vi "LIA Example FPGA_v1.vi"() -> ()   [LabVIEW 2017]
uses:
  <instrlib>/_niInstr/Streaming/v1/Common/Stream State.ctl
  <instrlib>/_niInstr/Data Trigger/v1/Shared/Public/Edge Configuration FXP(+-,18,1).ctl
  <instrlib>/_niInstr/Data Trigger/v1/Shared/Public/Edge Configuration Trigger Slope.ctl
  <vilib>/Platform/TimedLoop/XDataNode/timing_clust.ctl
  <vilib>/Platform/TimedLoop/XDataNode/nitl_modes.ctl
  <vilib>/Platform/TimedLoop/XDataNode/wakeup.ctl
  <instrlib>/_niInstr/DSP/v1/Shared/Public/IQ Data.ctl
  <vilib>/rvi/Emulation/niFpgaSctlEmulationGetInTimedLoop.vi
  <vilib>/rvi/Emulation/niFpgaEmulationReportErrorSimple.vi
  <vilib>/rvi/Emulation/niFpgaGetClockAttributes.vi
  <vilib>/rvi/Emulation/niFpgaCriticalErrorInLSC.vi
  <instrlib>/_niInstr/DSP/v1/FPGA/Public/Sub VIs/Frequency Shift/Frequency Shift - 1 spc.vi
  <instrlib>/_niInstr/DSP/v1/FPGA/Public/Sub VIs/Fractional Decimator/Fractional Decimator - 1 spc - 2x oc.vi
  <userlib>/_NI Noise Generation IP/FPGA/Public/Low Level/AWGN FXP23x2.vi
  <instrlib>/_niInstr/DSP/v1/FPGA/Public/Sub VIs/Frequency Shift/Frequency Shift - 2 spc.vi
  <vilib>/rvi/eio/common/nirviEmuTemplateMethod_errors.vi
  <vilib>/Platform/TimedLoop/XDataNode/XDataNode.xnode
  <instrlib>/_niInstr/DSP/v1/Xnodes/Public/Frequency Shift/niInstr DSP v1 Frequency Shift FPGA.xnode
  <vilib>/rvi/FXPMathLib/FxpMul/XNode/nifxpmath_Multiplier.xnode
  <vilib>/rvi/FXPMathLib/FxpAdd/XNode/nifxpmath_Add.xnode
  <vilib>/eio/EIONode/EIONode.xnode
  <vilib>/Platform/TimedLoop/XDataNode/XDNodeRunTimeDep.lvlib
  <instrlib>/_niInstr/Basic Elements/v1/FPGA/niInstr Basic Elements v1 FPGA.lvlib
  <instrlib>/_niInstr/DSP/v1/Shared/niInstr DSP v1 Shared.lvlib
  <instrlib>/_niInstr/DSP/v1/FPGA/niInstr DSP v1 FPGA.lvlib
  lib/fpga/Lock-In Amplifier Example FPGA.lvlib
  <instrlib>/_niInstr/Streaming/v1/Common/niInstr Streaming v1 Common.lvlib
  <userlib>/_NI Noise Generation IP/FPGA/NI Noise Generation IP FPGA v2.lvlib
  <vilib>/rvi/FXPMathLib/sim/FxpSim.dll
  <instrlib>/_niInstr/Data Trigger/v1/Shared/niInstr Data Trigger v1 Shared.lvlib
panel:
  in  "Decimator":enum16{"CIC", "FIR", "Bypassed"}(ring)
  in  "output sample rate":fxp<+,48,1>=0.0009999999999976694
  in  "pll.digital config 1":T1
  in  "pll.digital config 0":T1
  in  "pll.m 0":i8
  in  "pll.m 1":i8
  in  "pll.q 1":fxp<+,48,0>
  in  "pll.q 0":fxp<+,48,0>
  in  "lock-in.enable 3":bool
  in  "lock-in.enable 2":bool
  in  "lock-in.enable 1":bool
  in  "lock-in.carrier 3":fxp<+/-,48,0>
  in  "lock-in.carrier 2":fxp<+/-,48,0>
  in  "lock-in.enable 0":bool
  in  "lock-in.channel select 3":i32
  in  "lock-in.carrier select 3":i32
  in  "lock-in.cic config valid 3":bool
  in  "lock-in.cic config 3":cluster{"factor":fxp<+,16,16>, "shift":i16}
  in  "lock-in.reset 3":bool
  out "stream.state 3":T3 caption="stream.state 0"
  out "stream.samples transferred 3":u64 caption="stream.samples transferred 0"
  out "stream.metadata 3":u64 caption="stream.metadata 0"
  in  "stream.num samples 3":u64 caption="stream.num samples 0"
  in  "stream.request state 3":T3 caption="stream.request state 0"
  in  "lock-in.channel select 2":i32
  in  "lock-in.carrier select 2":i32
  in  "lock-in.cic config valid 2":bool
  in  "lock-in.cic config 2":cluster{"factor":fxp<+,16,16>, "shift":i16}
  in  "lock-in.reset 2":bool
  out "stream.state 2":T3 caption="stream.state 0"
  out "stream.samples transferred 2":u64 caption="stream.samples transferred 0"
  out "stream.metadata 2":u64 caption="stream.metadata 0"
  in  "stream.num samples 2":u64 caption="stream.num samples 0"
  in  "stream.request state 2":T3 caption="stream.request state 0"
  out "pll.vco output 0":fxp<+/-,48,0> format="%.49g"
  out "pll.vco output 1":fxp<+/-,48,0> format="%.49g"
  out "stream.metadata 4":u64 caption="stream.metadata 0"
  out "stream.samples transferred 4":u64 caption="stream.samples transferred 0"
  out "stream.state 4":T3 caption="stream.state 0"
  in  "stream.request state 4":T3 caption="stream.request state 0"
  in  "stream.num samples 4":u64 caption="stream.num samples 0"
  in  "preview.channel select":i32
  in  "ao.reset 3":bool
  in  "ao.carrier 2":fxp<+/-,48,0>=0.010000000000001563
  in  "ao.level 2":fxp<+/-,18,1>
  in  "ao.reset 2":bool
  in  "ao.carrier 1":fxp<+/-,48,0>=0.010000000000001563
  in  "ao.level 1":fxp<+/-,18,1>
  in  "ao.reset 1":bool
  in  "ao.reset 0":bool
  in  "ao.carrier 0":fxp<+/-,48,0>=0.010000000000001563
  in  "ao.level 0":fxp<+/-,18,1>
  in  "lock-in.channel select 1":i32
  in  "lock-in.channel select 0":i32
  in  "stream.request state 1":T3 caption="stream.request state 0"
  in  "stream.num samples 1":u64 caption="stream.num samples 0"
  out "stream.metadata 1":u64 caption="stream.metadata 0"
  out "stream.samples transferred 1":u64 caption="stream.samples transferred 0"
  out "stream.state 1":T3 caption="stream.state 0"
  in  "lock-in.reset 1":bool
  in  "lock-in.cic config 1":cluster{"factor":fxp<+,16,16>, "shift":i16}
  in  "lock-in.cic config valid 1":bool
  in  "lock-in.carrier select 1":i32
  in  "lock-in.carrier select 0":i32
  in  "lock-in.cic config valid 0":bool
  in  "lock-in.cic config 0":cluster{"factor":fxp<+,16,16>, "shift":i16}
  in  "lock-in.reset 0":bool
  in  "lock-in.carrier 1":fxp<+/-,48,0>
  in  "lock-in.carrier 0":fxp<+/-,48,0>
  in  "ao.level 3":fxp<+/-,18,1>
  in  "pll.channel 1":i32
  in  "pll.reset 1":bool
  in  "pll.enable 1":bool
  in  "pll.channel 0":i32
  in  "ao.noise gain 3":fxp<+,18,1>=0.01000213623046875
  in  "ao.carrier 3":fxp<+/-,48,0>=0.010000000000001563
  in  "ao.noise seeds 3":fxp<+,23,23>[](array[numeric])=[1.0, 12323.0]
  in  "pll.reset 0":bool
  in  "pll.enable 0":bool
  in  "stream.request state 0":T3
  in  "stream.num samples 0":u64
  out "stream.metadata 0":u64
  out "stream.samples transferred 0":u64
  out "stream.state 0":T3
  out "IO Module\\InitDone":bool
  out "IO Module\\User Error":u32
  in  "IO Module\\User Command":u32
  in  "IO Module\\User Command Valid":bool
  out "IO Module\\User Command Ready":bool
  in  "IO Module\\User Command Arg 0":u32
  in  "IO Module\\User Command Arg 1":u32
  out "IO Module\\User Command Error":u16
  out "IO Module\\User Command Return":u32
  out "IO Module\\User Command Return Valid":bool
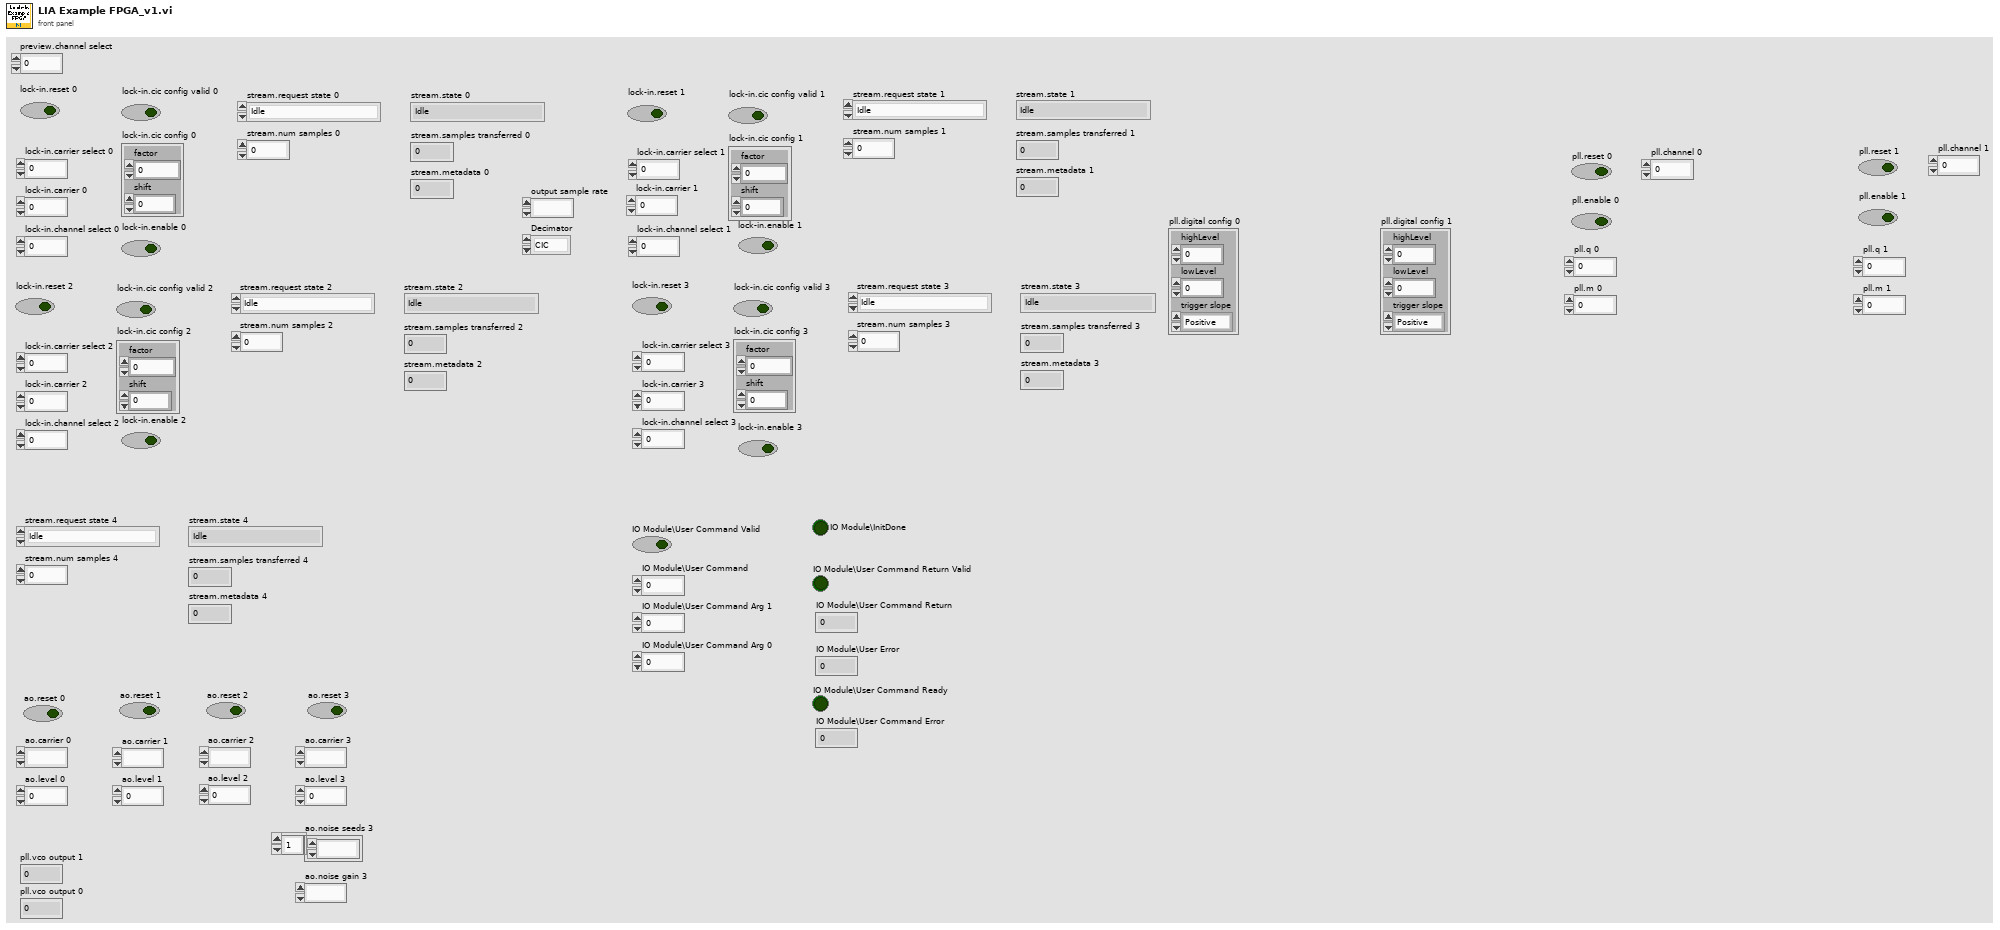
[diagram p1: front panel]
types:
  T1 = typedef "niInstr Data Trigger v1 Shared.lvlib/Edge Configuration FXP(+-,18,1).ctl" = cluster{"highLevel":fxp<+/-,18,1>, "lowLevel":fxp<+/-,18,1>, "trigger slope":T2}
  T2 = typedef "niInstr Data Trigger v1 Shared.lvlib/Edge Configuration Trigger Slope.ctl" = enum8{"Positive", "Negative"}
  T3 = typedef "niInstr Streaming v1 Common.lvlib/Stream State.ctl" = enum8{"Idle", "Finite Transfer", "Continuous", "Done", "Error", "Not Ready", "Cancel"}
  T4 = typedef "XDNodeRunTimeDep.lvlib/timing_clust.ctl" = cluster{"Expected End [f-1]":u64, "Actual End [f-1]":u64, "Finished Late? [f-1]":bool, "Expected End [i-1]":u64, "Actual End [i-1]":u64, "Finished Late? [i-1]":bool, "Expected Start [i]":u64, "Actual Start [i]":u64, "Expected Start [f]":u64, "Actual Start [f]":u64, "Source Name":string, "Structure Name":string, "Period":i64, "Deadline":i64, "Offset":i64, "Start":i64, "Priority":i32, "Timeout":i32, "Mode":T5, "Wakeup Reason":T6, "Error":errorcluster, "Source Type":string, "Secondary Source Type":string, "Global End Time":u64, "Global Start Time":u64, "Frame Duration":u64, "Iteration Duration":u64, "Assigned CPU":i32, "I/O Scan Engine Mode":u32}
  T5 = typedef "XDNodeRunTimeDep.lvlib/nitl_modes.ctl" = enum32{"No Change", "Process missed periods, maintain original phase", "Discard missed periods, maintain original phase", "Process missed periods, ignore original phase", "Discard missed periods, ignore original phase"}
  T6 = typedef "XDNodeRunTimeDep.lvlib/wakeup.ctl" = enum32{"Normal", "Aborted", "Asynchronous wakeup", "Timing source error", "Timed loop error", "Timeout"}
  T7 = cluster{"stream.num samples 0":u64, "stream.request state 0":T3, "stream.index 0":i16}
  T8 = typedef "niInstr DSP v1 Shared.lvlib/IQ Data.ctl" = cluster{"I":fxp<+/-,18,1>, "Q":fxp<+/-,18,1>, "overflow":bool}
  T9 = cluster{"stream.metadata 0":u64, "stream.samples transferred 0":u64, "stream.state 0":T3}
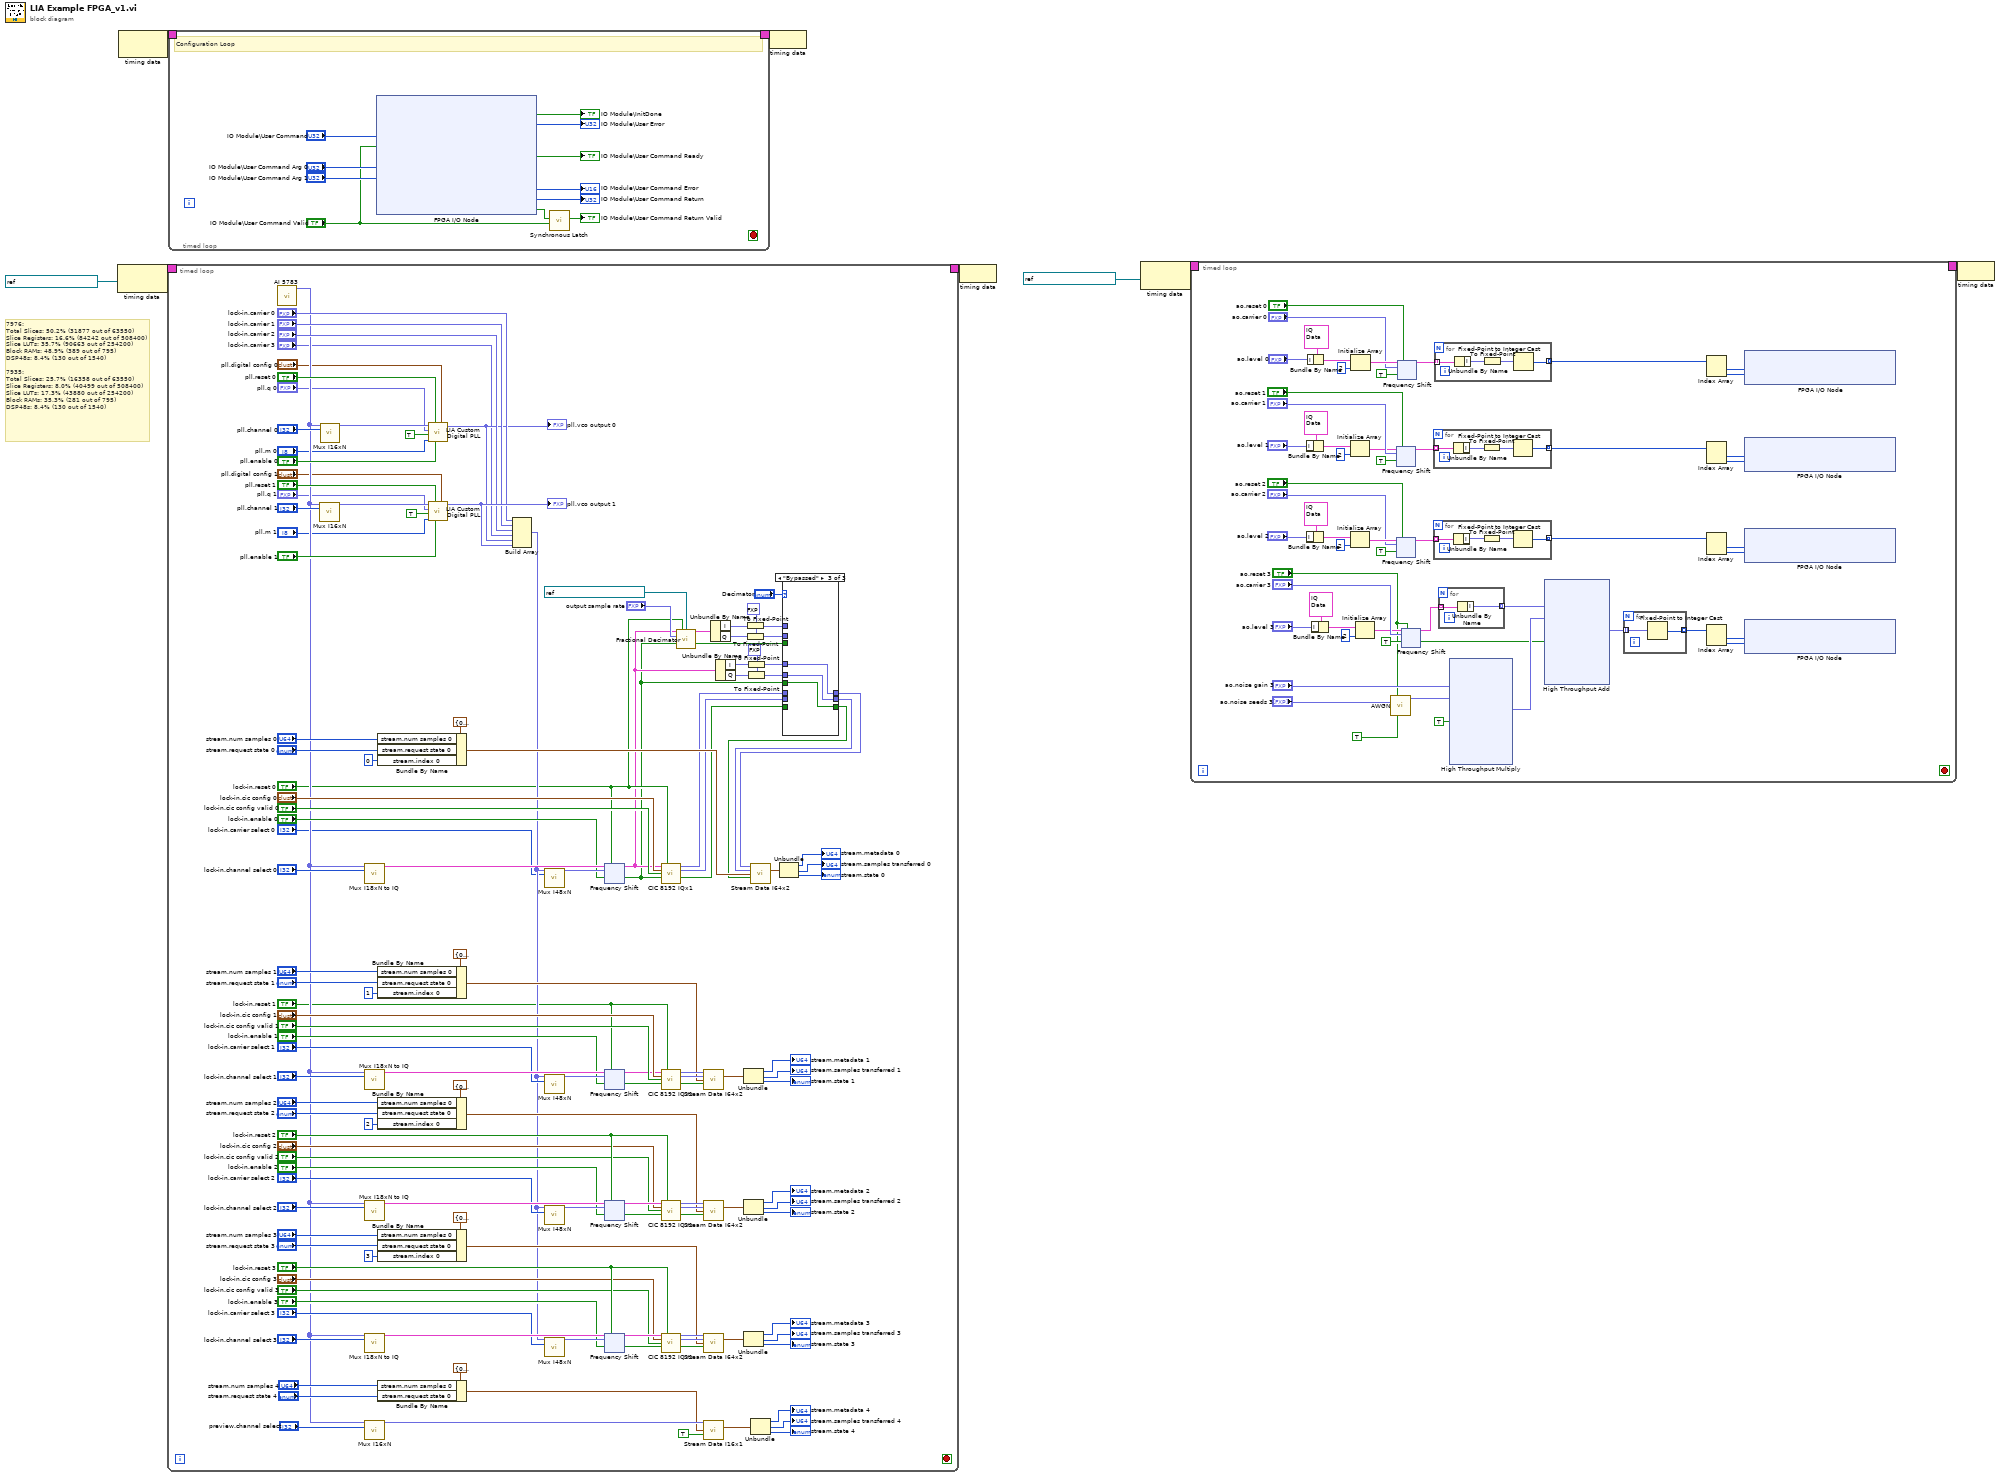
[diagram p0: block diagram]
diagram:
  # "7976:\nTotal Slices: 50.2% (31877 out of 63550)\nSlice Registers: 16.6% (84242 out of 508400)\nSlice LUTs: 35.7% (90663 out of 254200)\nBlock RAMs: 48.9% (389 out of 795)\nDSP48s: 8.4% (130 out of 1540)\n\n7935:\nTotal Slices: 25.7% (16358 out of 63550)\nSlice Registers: 8.0% (40499 out of 508400)\nSlice LUTs: 17.3% (43880 out of 254200)\nBlock RAMs: 35.3% (281 out of 795)\nDSP48s: 8.4% (130 out of 1540)"
  n1 = node-c288(refnum<k21> "IO Module\\Data Clock" ("Source Name")) -> (w8:T4)
  n2 = node-c288() -> (w2:T4)  [unwired: 1 in]
  n3 = timed-loop {
    timing: w8 -> [_]
    timing-out: [_] -> w7
    stop <- _ stop-if-true
    w13 = fxp<+/-,64,1> 0.0 ("i out")
    w27 = fxp<+/-,64,1> 0.0 ("i out")
    n4 = call "AI 5783.vi"() -> ("i18x1"=w45:fxp<+/-,18,1>[])  [unwired: 14 in, 1 out]
    n5 = call "Mux I16xN.vi"("i16xn in"=w45, "index"="pll.channel 1") -> ("i16 out"=w48:fxp<+/-,18,1>)  [unwired: 12 in, 1 out]
    n6 = call "Mux I16xN.vi"("i16xn in"=w45, "index"="pll.channel 0") -> ("i16 out"=w147:fxp<+/-,18,1>)  [unwired: 12 in, 1 out]
    n7 = call "Mux I18xN to IQ.vi"("i16xn in"=w45, "index"="lock-in.channel select 0") -> ("output"=w142:T8)  [unwired: 12 in, 1 out]
    n8 = call "Mux I18xN to IQ.vi"("i16xn in"=w45, "index"="lock-in.channel select 1") -> ("output"=w128:T8)  [unwired: 12 in, 1 out]
    n9 = call "Mux I18xN to IQ.vi"("i16xn in"=w45, "index"="lock-in.channel select 2") -> ("output"=w99:T8)  [unwired: 12 in, 1 out]
    n10 = call "Mux I18xN to IQ.vi"("i16xn in"=w45, "index"="lock-in.channel select 3") -> ("output"=w78:T8)  [unwired: 12 in, 1 out]
    n11 = call "Mux I16xN.vi"("i16xn in"=w45, "index"="preview.channel select") -> ("i16 out"=w105:fxp<+/-,18,1>)  [unwired: 12 in, 1 out]
    n12 = Bundle By Name(cluster=T7 {"stream.num samples 0"=0, "stream.request state 0"=enum."Idle", "stream.index 0"=0} ("config"), "stream.num samples 0"="stream.num samples 0", "stream.request state 0"="stream.request state 0", "stream.index 0"=i16 0) -> (w130:T7)
    n13 = Bundle By Name(cluster=T7 {"stream.num samples 0"=0, "stream.request state 0"=enum."Idle", "stream.index 0"=0} ("config"), "stream.num samples 0"="stream.num samples 1", "stream.request state 0"="stream.request state 1", "stream.index 0"=i16 1) -> (w113:T7)
    n14 = Bundle By Name(cluster=T7 {"stream.num samples 0"=0, "stream.request state 0"=enum."Idle", "stream.index 0"=0} ("config"), "stream.num samples 0"="stream.num samples 2", "stream.request state 0"="stream.request state 2", "stream.index 0"=i16 2) -> (w81:T7)
    n15 = Bundle By Name(cluster=T7 {"stream.num samples 0"=0, "stream.request state 0"=enum."Idle", "stream.index 0"=0} ("config"), "stream.num samples 0"="stream.num samples 3", "stream.request state 0"="stream.request state 3", "stream.index 0"=i16 3) -> (w60:T7)
    n16 = Bundle By Name(cluster=T7 {"stream.num samples 0"=0, "stream.request state 0"=enum."Idle", "stream.index 0"=0} ("config"), "stream.num samples 0"="stream.num samples 4", "stream.request state 0"="stream.request state 4") -> (w102:T7)
    n17 = call "LIA Custom Digital PLL.vi"("configuration"="pll.digital config 0", "arm"="pll.enable 0", "reset"="pll.reset 0", "m"="pll.m 0", "input valid"=TRUE ("output valid"), "q"="pll.q 0", "I"=w147) -> ("frequency shift"=w47:fxp<+/-,48,0>)  [unwired: 1 in, 3 out]
    "pll.vco output 0" <- w47
    n18 = call "LIA Custom Digital PLL.vi"("configuration"="pll.digital config 1", "arm"="pll.enable 1", "reset"="pll.reset 1", "m"="pll.m 1", "input valid"=TRUE ("output valid"), "q"="pll.q 1", "I"=w48) -> ("frequency shift"=w100:fxp<+/-,48,0>)  [unwired: 1 in, 3 out]
    "pll.vco output 1" <- w100
    n19 = Build Array("lock-in.carrier 0", "lock-in.carrier 1", "lock-in.carrier 2", "lock-in.carrier 3", w47, w100) -> (w46:fxp<+/-,48,0>[])
    n20 = call "Mux I48xN.vi"("i48xn in"=w46, "index"="lock-in.carrier select 0") -> ("i48 out"=w141:fxp<+/-,48,0>)  [unwired: 13 in]
    n21 = call "Mux I48xN.vi"("i48xn in"=w46, "index"="lock-in.carrier select 1") -> ("i48 out"=w127:fxp<+/-,48,0>)  [unwired: 13 in]
    n22 = call "Mux I48xN.vi"("i48xn in"=w46, "index"="lock-in.carrier select 2") -> ("i48 out"=w98:fxp<+/-,48,0>)  [unwired: 13 in]
    n23 = call "Mux I48xN.vi"("i48xn in"=w46, "index"="lock-in.carrier select 3") -> ("i48 out"=w77:fxp<+/-,48,0>)  [unwired: 13 in]
    n24 = xnode "Frequency Shift"("data in"=w142, "reset"="lock-in.reset 0", "frequency shift"=w141, "input valid"="lock-in.enable 0") -> ("data out"=w12:T8, "output valid"=w9:bool)  [unwired: 2 in, 1 out]
    n25 = xnode "Frequency Shift"("data in"=w128, "reset"="lock-in.reset 1", "frequency shift"=w127, "input valid"="lock-in.enable 1") -> ("data out"=w34:T8, "output valid"=w32:bool)  [unwired: 2 in, 1 out]
    n26 = xnode "Frequency Shift"("data in"=w99, "reset"="lock-in.reset 2", "frequency shift"=w98, "input valid"="lock-in.enable 2") -> ("data out"=w97:T8, "output valid"=w96:bool)  [unwired: 2 in, 1 out]
    n27 = xnode "Frequency Shift"("data in"=w78, "reset"="lock-in.reset 3", "frequency shift"=w77, "input valid"="lock-in.enable 3") -> ("data out"=w76:T8, "output valid"=w75:bool)  [unwired: 2 in, 1 out]
    n28 = call "CIC 8192 IQx1.vi"("data"=w12, "reset"="lock-in.reset 0", "config"="lock-in.cic config 0", "config valid"="lock-in.cic config valid 0", "input valid"=w9) -> ("i out"=w19:fxp<+/-,64,1>, "q out"=w21:fxp<+/-,64,1>, "output valid"=w24:bool)  [unwired: 8 in]
    n29 = call "CIC 8192 IQx1.vi"("data"=w34, "reset"="lock-in.reset 1", "config"="lock-in.cic config 1", "config valid"="lock-in.cic config valid 1", "input valid"=w32) -> ("i out"=w124:fxp<+/-,64,1>, "q out"=w123:fxp<+/-,64,1>, "output valid"=w122:bool)  [unwired: 8 in]
    n30 = call "CIC 8192 IQx1.vi"("data"=w97, "reset"="lock-in.reset 2", "config"="lock-in.cic config 2", "config valid"="lock-in.cic config valid 2", "input valid"=w96) -> ("i out"=w92:fxp<+/-,64,1>, "q out"=w91:fxp<+/-,64,1>, "output valid"=w90:bool)  [unwired: 8 in]
    n31 = call "CIC 8192 IQx1.vi"("data"=w76, "reset"="lock-in.reset 3", "config"="lock-in.cic config 3", "config valid"="lock-in.cic config valid 3", "input valid"=w75) -> ("i out"=w71:fxp<+/-,64,1>, "q out"=w70:fxp<+/-,64,1>, "output valid"=w69:bool)  [unwired: 8 in]
    n32 = call-poly <instrlib>:"Fractional Decimator.vi"("data in"=w12, "reset"="lock-in.reset 0", "clock x 2"=refnum<k21> "IO Module\\Data Clock 2x", "output sample rate"="output sample rate", "input valid"=w9) -> ("data out"=w30:T8, "output valid"=w18:bool)  [unwired: 8 in, 1 out]
    n33 = call "Stream Data I64x2.vi"("i in"=w124, "q in"=w123, "config"=w113, "input valid"=w122) -> ("status"=w121:T9)  [unwired: 11 in]
    n34 = call "Stream Data I64x2.vi"("i in"=w92, "q in"=w91, "config"=w81, "input valid"=w90) -> ("status"=w89:T9)  [unwired: 11 in]
    n35 = call "Stream Data I64x2.vi"("i in"=w71, "q in"=w70, "config"=w60, "input valid"=w69) -> ("status"=w68:T9)  [unwired: 11 in]
    n36 = call "Stream Data I16x1.vi"("i in"=w105, "config"=w102, "input valid"=TRUE) -> ("status"=w107:T9)  [unwired: 12 in]
    n37 = Unbundle By Name(w30) -> ("I"=w29:fxp<+/-,18,1>, "Q"=w28:fxp<+/-,18,1>)
    n38 = Unbundle By Name(w12) -> ("I"=w14:fxp<+/-,18,1>, "Q"=w15:fxp<+/-,18,1>)
    n39 = Unbundle(w121) -> ("stream.metadata 0"=→"stream.metadata 1":u64, "stream.samples transferred 0"=→"stream.samples transferred 1":u64, "stream.state 0"=→"stream.state 1":T3)
    n40 = Unbundle(w89) -> ("stream.metadata 0"=→"stream.metadata 2":u64, "stream.samples transferred 0"=→"stream.samples transferred 2":u64, "stream.state 0"=→"stream.state 2":T3)
    n41 = Unbundle(w68) -> ("stream.metadata 0"=→"stream.metadata 3":u64, "stream.samples transferred 0"=→"stream.samples transferred 3":u64, "stream.state 0"=→"stream.state 3":T3)
    n42 = To Fixed-Point(fixed-point type=w27, number=w29) -> (fixed-point=w16:fxp<+/-,64,1>)
    n43 = To Fixed-Point(fixed-point type=w27, number=w28) -> (fixed-point=w17:fxp<+/-,64,1>)
    n44 = To Fixed-Point(fixed-point type=w13, number=w14) -> (fixed-point=w11:fxp<+/-,64,1>)
    n45 = To Fixed-Point(fixed-point type=w13, number=w15) -> (fixed-point=w10:fxp<+/-,64,1>)
    n46 = Unbundle(w107) -> ("stream.metadata 0"=→"stream.metadata 4":u64, "stream.samples transferred 0"=→"stream.samples transferred 4":u64, "stream.state 0"=→"stream.state 4":T3)
    n47 = case shown="\"Bypassed\"" "Decimator" {
      tunnel: w24 -> [w152 _ _]
      tunnel: [w152 w155 w156] -> w23
      tunnel: [w151 w154 w157] -> w22
      tunnel: w21 -> [w151 _ _]
      tunnel: [w150 w153 w158] -> w20
      tunnel: w19 -> [w150 _ _]
      tunnel: w18 -> [_ w155 _]
      tunnel: w17 -> [_ w154 _]
      tunnel: w16 -> [_ w153 _]
      tunnel: w11 -> [_ _ w158]
      tunnel: w10 -> [_ _ w157]
      tunnel: w9 -> [_ _ w156]
      frame "CIC", Default {
      }
      frame "FIR" {
      }
      frame "Bypassed" {
      }
    }
    n48 = call "Stream Data I64x2.vi"("i in"=w20, "q in"=w22, "config"=w130, "input valid"=w23) -> ("status"=w138:T9)  [unwired: 11 in]
    n49 = Unbundle(w138) -> ("stream.metadata 0"=→"stream.metadata 0":u64, "stream.samples transferred 0"=→"stream.samples transferred 0":u64, "stream.state 0"=→"stream.state 0":T3)
  }
  n50 = timed-loop {
    timing: w2 -> [_]
    timing-out: [_] -> w1
    stop <- _ stop-if-true
    # "Configuration Loop"
    n51 = xnode "FPGA I/O Node"("IO Module\\User Command"="IO Module\\User Command", "IO Module\\User Command Valid"="IO Module\\User Command Valid", "IO Module\\User Command Arg 0"="IO Module\\User Command Arg 0", "IO Module\\User Command Arg 1"="IO Module\\User Command Arg 1") -> ("IO Module\\InitDone"=→"IO Module\\InitDone":bool, "IO Module\\Clip Error Code"=→"IO Module\\User Error":u32, "IO Module\\User Command Ready"=→"IO Module\\User Command Ready":bool, "IO Module\\User Command Error"=→"IO Module\\User Command Error":u16, "IO Module\\User Command Return"=→"IO Module\\User Command Return":u32, "IO Module\\User Command Return Valid"=w198:bool)  [unwired: 10 in, 10 out]
    n52 = call <instrlib>:"Synchronous Latch.vi"("clear"="IO Module\\User Command Valid", "set"=w198) -> ("out"=→"IO Module\\User Command Return Valid":bool)  [unwired: 9 in]
  }
  n53 = node-c288(w1) -> ()
  n54 = node-c288(w7) -> ()
  n55 = node-c288(refnum<k21> "IO Module\\Data Clock" ("Source Name")) -> (w5:T4)
  n56 = timed-loop {
    timing: w5 -> [_]
    timing-out: [_] -> w4
    stop <- _ stop-if-true
    n57 = Bundle By Name(cluster=T8 {"I"=0.0, "Q"=0.0, "overflow"=FALSE} ("output"), "I"="ao.level 1") -> (w231:T8)
    n58 = Bundle By Name(cluster=T8 {"I"=0.0, "Q"=0.0, "overflow"=FALSE} ("output"), "I"="ao.level 2") -> (w221:T8)
    n59 = Bundle By Name(cluster=T8 {"I"=0.0, "Q"=0.0, "overflow"=FALSE} ("output"), "I"="ao.level 0") -> (w246:T8)
    n60 = Bundle By Name(cluster=T8 {"I"=0.0, "Q"=0.0, "overflow"=FALSE} ("output"), "I"="ao.level 3") -> (w255:T8)
    n61 = Initialize Array(w231, 2 ("dimension size")) -> (w227:T8[])
    n62 = Initialize Array(w221, 2 ("dimension size")) -> (w225:T8[])
    n63 = Initialize Array(w246, 2 ("dimension size")) -> (w250:T8[])
    n64 = Initialize Array(w255, 2 ("dimension size")) -> (w251:T8[])
    n65 = call-poly <userlib>:"AWGN.vi"("reset"="ao.reset 3", "seeds"="ao.noise seeds 3", "ready"=TRUE) -> ("output 0"=w258:fxp<+/-,23,4>[])  [unwired: 10 in, 2 out]
    n66 = xnode "Frequency Shift"("data in"=w227, "reset"="ao.reset 1", "frequency shift"="ao.carrier 1", "input valid"=TRUE) -> ("data out"=w235:T8[])  [unwired: 2 in, 2 out]
    n67 = xnode "Frequency Shift"("data in"=w225, "reset"="ao.reset 2", "frequency shift"="ao.carrier 2", "input valid"=TRUE) -> ("data out"=w217:T8[])  [unwired: 2 in, 2 out]
    n68 = xnode "Frequency Shift"("data in"=w250, "reset"="ao.reset 0", "frequency shift"="ao.carrier 0", "input valid"=TRUE) -> ("data out"=w242:T8[])  [unwired: 2 in, 2 out]
    n69 = xnode "Frequency Shift"("data in"=w251, "reset"="ao.reset 3", "frequency shift"="ao.carrier 3", "input valid"=TRUE) -> ("data out"=w266:T8[], "output valid"=w263:bool)  [unwired: 2 in, 1 out]
    n70 = for {
      tunnel: w235 -> [w282] mode=indexing
      tunnel: [w283] -> w236 mode=indexing
      n71 = Unbundle By Name(w282) -> ("I"=w281:fxp<+/-,18,1>)
      n72 = To Fixed-Point(number=w281) -> (fixed-point=w280:fxp<+/-,16,1>)  [unwired: 1 in]
      n73 = Fixed-Point to Integer Cast(1:w280) -> (0:w283:i16)
    }
    n74 = for {
      tunnel: w217 -> [w269] mode=indexing
      tunnel: [w270] -> w216 mode=indexing
      n75 = Unbundle By Name(w269) -> ("I"=w268:fxp<+/-,18,1>)
      n76 = To Fixed-Point(number=w268) -> (fixed-point=w267:fxp<+/-,16,1>)  [unwired: 1 in]
      n77 = Fixed-Point to Integer Cast(1:w267) -> (0:w270:i16)
    }
    n78 = for {
      tunnel: w242 -> [w295] mode=indexing
      tunnel: [w296] -> w241 mode=indexing
      n79 = Unbundle By Name(w295) -> ("I"=w294:fxp<+/-,18,1>)
      n80 = To Fixed-Point(number=w294) -> (fixed-point=w293:fxp<+/-,16,1>)  [unwired: 1 in]
      n81 = Fixed-Point to Integer Cast(1:w293) -> (0:w296:i16)
    }
    n82 = for {
      tunnel: w266 -> [w309] mode=indexing
      tunnel: [w308] -> w262 mode=indexing
      n83 = Unbundle By Name(w309) -> ("I"=w308:fxp<+/-,18,1>)
    }
    n84 = xnode ("High Throughput Multiply")("x"="ao.noise gain 3", "y"=w258, "input valid"=TRUE) -> ("x*y"=w265:fxp<+/-,41,5>[])  [unwired: 1 in, 2 out]
    n85 = xnode ("High Throughput Add")("x"=w262, "y"=w265, "input valid"=w263) -> ("x+y"=w257:fxp<+/-,16,1>[])  [unwired: 1 in, 2 out]
    n86 = for {
      tunnel: w257 -> [w307] mode=indexing
      tunnel: [w306] -> w226 mode=indexing
      n87 = Fixed-Point to Integer Cast(1:w307) -> (0:w306:i16)
    }
    n88 = Index Array(array=w241) -> (element #1=w240:i16, element #2=w239:i16)  [unwired: 2 in]
    n89 = Index Array(array=w236) -> (element #1=w237:i16, element #2=w238:i16)  [unwired: 2 in]
    n90 = Index Array(array=w216) -> (element #1=w215:i16, element #2=w214:i16)  [unwired: 2 in]
    n91 = Index Array(array=w226) -> (element #1=w213:i16, element #2=w212:i16)  [unwired: 2 in]
    n92 = xnode "FPGA I/O Node"("IO Module\\AO 1 Data N-1 Data Clock"=w237, "IO Module\\AO 1 Data N Data Clock"=w238) -> ()  [unwired: 2 in, 2 out]
    n93 = xnode "FPGA I/O Node"("IO Module\\AO 2 Data N-1 Data Clock"=w215, "IO Module\\AO 2 Data N Data Clock"=w214) -> ()  [unwired: 2 in, 2 out]
    n94 = xnode "FPGA I/O Node"("IO Module\\AO 3 Data N-1 Data Clock"=w213, "IO Module\\AO 3 Data N Data Clock"=w212) -> ()  [unwired: 2 in, 2 out]
    n95 = xnode "FPGA I/O Node"("IO Module\\AO 0 Data N-1 Data Clock"=w240, "IO Module\\AO 0 Data N Data Clock"=w239) -> ()  [unwired: 2 in, 2 out]
  }
  n96 = node-c288(w4) -> ()
